vi "Open Existing Buffer.vi"(8 "error in (no error)":errorcluster, 9 "timeout (ms)":i32=2000, 11 "buffer_name":string="/example") -> (0 "error out":errorcluster, 3 "CIPC Reference":u64)   [LabVIEW 2021, in "CIF_NI_CIPC.lvlib"]
doc: "Open an existing CIPC buffer.s\n\nInputs:\n- buffer_name: name of the buffer\n- timeout: timeout in ms to wait for the CIPC buffer to be created.\n- prepend array or string size?: if true, the elements in the buffer will have their array size prepended in the data\n\nOutputs:\n- buffer_refs: reference and information on the created/opened CIPC buffer\ns"
uses:
  CIF_NI_CIPC.lvlib
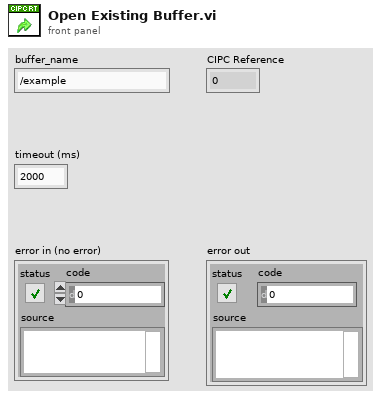
[diagram p1: front panel]
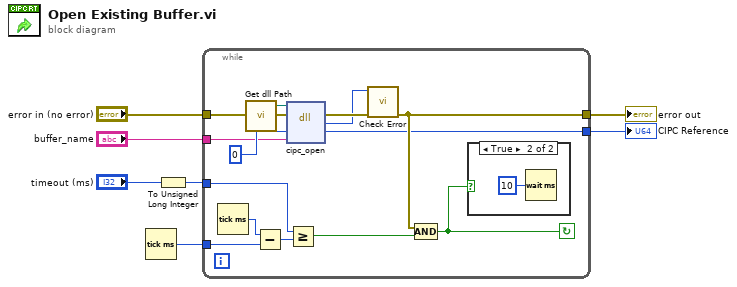
[diagram p0: block diagram]
diagram:
  n1 = Tick Count (ms)() -> (millisecond timer value=w7:u32)
  n2 = To Unsigned Long Integer(number="timeout (ms)") -> (unsigned 32bit integer=w5:u32)
  n3 = while {
    tunnel: [w12] -> w1
    tunnel: w7 -> [w17]
    tunnel: w5 -> [w15]
    tunnel: "buffer_name" -> [w13]
    tunnel: "error in (no error)" -> [w11]
    tunnel: [w10] -> w2
    stop <- w9 continue-if-true
    n4 = Tick Count (ms)() -> (millisecond timer value=w18:u32)
    n5 = call "Get dll Path.vi"() -> ("appended path"=w8:path)  [unwired: 5 in]
    n6 = Subtract(x=w18, y=w17) -> (x-y=w14:u32)
    n7 = dll-call lib="libnicipc.*" fn="cipc_open"(path in=w8, error in=w11, "cipc_buffer_ref"=u64 0, "name"=w13) -> (error out=w20:errorcluster, "return type"=w19:i32, "cipc_buffer_ref"=w10:u64)  [unwired: 2 in, 1 out]
    n8 = Greater Or Equal?(x=w15, y=w14) -> (x >= y?=w16:bool)
    n9 = call "Check Error.vi"("error in (no error)"=w20, "Error Code"=w19) -> ("error out"=w12:errorcluster)  [unwired: 9 in]
    n10 = Compound Arithmetic op=AND(w12, w16) -> (w9:bool)
    n11 = case shown="True" w9 {
      frame False {
      }
      frame True {
        n12 = Wait (ms)(milliseconds to wait=u32 10) -> ()  [unwired: 1 out]
      }
    }
  }
  "error out" <- w1
  "CIPC Reference" <- w2
